vi "ReadFile.vi"(11 "UFF Path":path) -> (2 "transfer fct":cluster{"x0":dbl, "df":dbl, dbl[]}[](graph))   [LabVIEW 2024]
uses:
  PreferencesControl.ctl
panel:
  out "Header Info":T1
  out "Y":cdb[](array[numeric])
  out "Info 3":T2 {"Sampling Type" items=["Dynamic", "Static", "RPM from Tach", "Freq from Tach"]; "Z-axis Data Type Qualifier" items=["Translation", "Rotation", "Translation squared", "Rotation squared"]; "Ordinate Denominator Data Type Qualifier" items=["Translation", "Rotation", "Translation squared", "Rotation squared"]; "Ordinate Numerator Data Type Qualifier" items=["Translation", "Rotation", "Translation squared", "Rotation squared"]; "Abscissa Data Type Qualifier" items=["Translation", "Rotation", "Translation squared", "Rotation squared"]; "Normalization Method" items=["Unknown", "Units squared", "Units squared per Hz", "Units squared sec per Hz"]; "Amplitude units" items=["unknown", "Half-peak scale", "Peak scale", "RMS"]; "Window Type" items=["None", "Hanning Broad", "Hanning Narrow", "Flattop", "Exponential", "Impact", "Impact & Exponential"]; "Weighting Type" items=["None", "A weighting", "B weighting", "C weighting", "D weighting"]}
  out "Info 2":T3 {"Octave Format" items=["Not in octave format", "octave", "/12 octave", "one third octave", "1/n octave"]}
  out "Time n Type":T4={"Date"="Frequency", "Time"="Frequency", "Version from DB"=0.0, "Subversion"=0.0, "File Type"=enum."Universal"}
  out "Last Saved":cluster{"Date":string, "Time":string}={"Date"="Frequency", "Time"="Frequency"}
  out "Parent Program":string="Frequency"
  out "Info":T5
  out "Nodes":T6
  out "Units":T7
  out "Conversions":T8
  out "Data":T9(array[cluster]) {"Data"."dX" format="%#.6f"}
  out "Tracelines":T10 {"nodes defining" items=["move to node", "draw line to node"]}
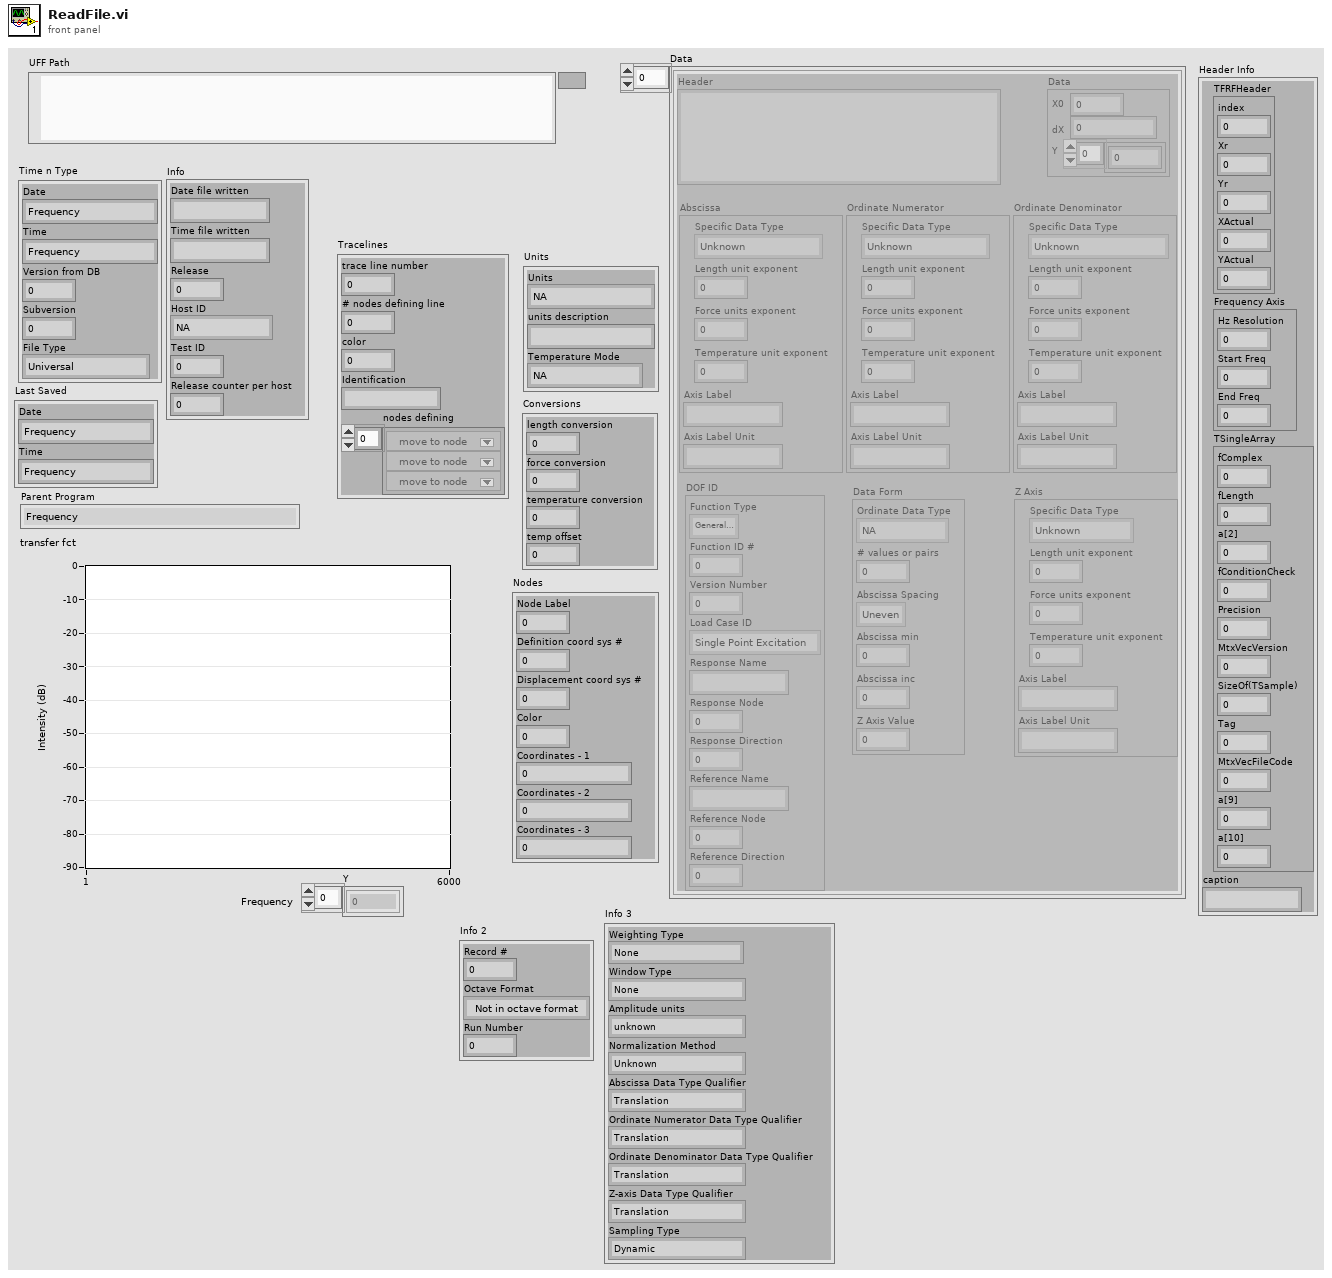
[diagram p1: front panel]
types:
  T1 = cluster{"TFRFHeader":cluster{"index":u32, "Xr":dbl, "Yr":dbl, "XActual":dbl, "YActual":dbl}, "Frequency Axis":cluster{"Hz Resolution":dbl, "Start Freq":dbl, "End Freq":dbl}, "TSingleArray":cluster{"fComplex":u32, "fLength":dbl, "a[2]":dbl, "fConditionCheck":dbl, "Precision":dbl, "MtxVecVersion":dbl, "SizeOf(TSample)":dbl, "Tag":dbl, "MtxVecFileCode":dbl, "a[9]":dbl, "a[10]":dbl}, "caption":string}
  T2 = cluster{"Weighting Type":u16, "Window Type":u16, "Amplitude units":u16, "Normalization Method":u16, "Abscissa Data Type Qualifier":u16, "Ordinate Numerator Data Type Qualifier":u16, "Ordinate Denominator Data Type Qualifier":u16, "Z-axis Data Type Qualifier":u16, "Sampling Type":u16}
  T3 = cluster{"Record #":dbl, "Octave Format":u16, "Run Number":dbl}
  T4 = cluster{"Date":string, "Time":string, "Version from DB":dbl, "Subversion":dbl, "File Type":enum16{"Universal", "Archive", "Other"}}
  T5 = cluster{"Date file written":string, "Time file written":string, "Release":i32, "Host ID":enum16{"NA", "VAX", "SGI", "HP", "RS", "Alp", "Sun", "Sony", "NEC", "Alop/OSF"}, "Test ID":i32, "Release counter per host":i32}
  T6 = cluster{"Node Label":dbl, "Definition coord sys #":dbl, "Displacement coord sys #":dbl, "Color":dbl, "Coordinates - 1":dbl, "Coordinates - 2":dbl, "Coordinates - 3":dbl}
  T7 = cluster{"Units":enum16{"NA", "SIL: Meter", "BG: Foot", "MG: Meter", "BA: Foot", "MM: millimeter", "CM: cm", "IN: inch", "GM: mm", "US: user defined", "MN: mm"}, "units description":string, "Temperature Mode":enum16{"NA", "absolute", "relaitve"}}
  T8 = cluster{"length conversion":dbl, "force conversion":dbl, "temperature conversion":dbl, "temp offset":dbl}
  T9 = cluster{"Abscissa":cluster{"Specific Data Type":enum16{"Unknown", "general", "stress", "strain", "na1", "temperature", "heat flux", "displacement", "na2", "reaction force", "na3", "velocity", "acceleration", "excitation force", "na4", "pressure", "mass", "time", "frequency", "rpm", "order", "sound pressure", "sound intensity", "sound power"}, "Length unit exponent":i32, "Force units exponent":i32, "Temperature unit exponent":i32, "Axis Label":string, "Axis Label Unit":string}, "Ordinate Numerator":cluster{"Specific Data Type":enum16{"Unknown", "general", "stress", "strain", "na1", "temperature", "heat flux", "displacement", "na2", "reaction force", "na3", "velocity", "acceleration", "excitation force", "na4", "pressure", "mass", "time", "frequency", "rpm", "order", "sound pressure", "sound intensity", "sound power"}, "Length unit exponent":i32, "Force units exponent":i32, "Temperature unit exponent":i32, "Axis Label":string, "Axis Label Unit":string}, "Ordinate Denominator":cluster{"Specific Data Type":enum16{"Unknown", "general", "stress", "strain", "na1", "temperature", "heat flux", "displacement", "na2", "reaction force", "na3", "velocity", "acceleration", "excitation force", "na4", "pressure", "mass", "time", "frequency", "rpm", "order", "sound pressure", "sound intensity", "sound power"}, "Length unit exponent":i32, "Force units exponent":i32, "Temperature unit exponent":i32, "Axis Label":string, "Axis Label Unit":string}, "Z Axis":cluster{"Specific Data Type":enum16{"Unknown", "general", "stress", "strain", "na1", "temperature", "heat flux", "displacement", "na2", "reaction force", "na3", "velocity", "acceleration", "excitation force", "na4", "pressure", "mass", "time", "frequency", "rpm", "order", "sound pressure", "sound intensity", "sound power"}, "Length unit exponent":i32, "Force units exponent":i32, "Temperature unit exponent":i32, "Axis Label":string, "Axis Label Unit":string}, "Data Form":cluster{"Ordinate Data Type":enum16{"NA", "NA2", "Real SGL", "NA3", "Real DBL", "Complex SGL", "Complex DBL"}, "# values or pairs":i32, "Abscissa Spacing":enum16{"Uneven", "Even"}, "Abscissa min":dbl, "Abscissa inc":dbl, "Z Axis Value":dbl}, "DOF ID":cluster{"Function Type":enum16{"General or Unknown", "Time Response", "Auto Spectrum", "Cross Spectrum", "FRF", "Transmissibility", "Coherence", "Auto Correlation", "Cross Correlation", "Power Spectral Density", "Energy Spectral Density Function", "Prob Density Function", "Spectrum", "Cumulative Freq Dist", "Peaks Valley", "Stress/Cycles", "Strain/Cycles", "Orbit", "Mode Indicator Funct", "Force Pattern", "Partial Power", "Partial Coherence", "Eigenvalue", "Eigenvector", "Shock Response Spectrum", "Finite Inpulse Response Filter", "Multiple Coherence", "Order Function", "Phase Compensation"}, "Function ID #":i32, "Version Number":i32, "Load Case ID":enum16{"Single Point Excitation"}, "Response Name":string, "Response Node":i32, "Response Direction":i8, "Reference Name":string, "Reference Node":i32, "Reference Direction":i8}, "Data":cluster{"X0":dbl, "dX":dbl, "Y":dbl[]}, "Header":string}[]
  T10 = cluster{"trace line number":i16, "# nodes defining line":i16, "color":i16, "Identification":string, "nodes defining":u16[]}
  T11 = typedef "PreferencesControl.ctl" = cluster{"Name of test":string, "Date":timestamp, "Location":string, "Template":string, "Soundcard":string, "resolution":u16, "Sampling rate":u16, "Ch1 Gain ":dbl, "Ch2 Gain":dbl, "Sample time (s)":dbl, "Pre-trigger (s)":dbl, "Hammer Threshold":dbl, "Positions":i16, "Taps/Position":i16, "Set Names":string, "Freq resolution":dbl, "Hammer cutoff":dbl, "Mic cutoff":dbl, "Double bounce ":dbl, "Hammer Cal":dbl, "dB Offset":dbl, "Accel Cal":dbl, "Vibrometer Cal":dbl, "Mic Cal":dbl, "Output":u16, "Voltage Cal":dbl, "Vibrometer Port":refnum<visa-resource-name>, "Range":u16, "High Pass":u16, "Bandwidth":u16, "X Range":cluster{"Minimum":dbl, "Maximum":dbl, "Increment":dbl, "Minor Increment":dbl, "Start":dbl}[], "Y Range":cluster{"Minimum":dbl, "Maximum":dbl, "Increment":dbl, "Minor Increment":dbl, "Start":dbl}[], "dB Spread":dbl, "Trigger":u16, "Ch_1":u8, "Ch_2":u8, "flip?":bool, "60Hz":bool, "Time offset":dbl, "Piezo Cal":dbl, "Default Notes":string}
  T12 = cluster{"Abscissa":cluster{"Specific Data Type":enum16{"Unknown", "general", "stress", "strain", "na1", "temperature", "heat flux", "displacement", "na2", "reaction force", "na3", "velocity", "acceleration", "excitation force", "na4", "pressure", "mass", "time", "frequency", "rpm", "order", "sound pressure", "sound intensity", "sound power"}, "Length unit exponent":i32, "Force units exponent":i32, "Temperature unit exponent":i32, "Axis Label":string, "Axis Label Unit":string}, "Ordinate Numerator":cluster{"Specific Data Type":enum16{"Unknown", "general", "stress", "strain", "na1", "temperature", "heat flux", "displacement", "na2", "reaction force", "na3", "velocity", "acceleration", "excitation force", "na4", "pressure", "mass", "time", "frequency", "rpm", "order", "sound pressure", "sound intensity", "sound power"}, "Length unit exponent":i32, "Force units exponent":i32, "Temperature unit exponent":i32, "Axis Label":string, "Axis Label Unit":string}, "Ordinate Denominator":cluster{"Specific Data Type":enum16{"Unknown", "general", "stress", "strain", "na1", "temperature", "heat flux", "displacement", "na2", "reaction force", "na3", "velocity", "acceleration", "excitation force", "na4", "pressure", "mass", "time", "frequency", "rpm", "order", "sound pressure", "sound intensity", "sound power"}, "Length unit exponent":i32, "Force units exponent":i32, "Temperature unit exponent":i32, "Axis Label":string, "Axis Label Unit":string}, "Z Axis":cluster{"Specific Data Type":enum16{"Unknown", "general", "stress", "strain", "na1", "temperature", "heat flux", "displacement", "na2", "reaction force", "na3", "velocity", "acceleration", "excitation force", "na4", "pressure", "mass", "time", "frequency", "rpm", "order", "sound pressure", "sound intensity", "sound power"}, "Length unit exponent":i32, "Force units exponent":i32, "Temperature unit exponent":i32, "Axis Label":string, "Axis Label Unit":string}, "Data Form":cluster{"Ordinate Data Type":enum16{"NA", "NA2", "Real SGL", "NA3", "Real DBL", "Complex SGL", "Complex DBL"}, "# values or pairs":i32, "Abscissa Spacing":enum16{"Uneven", "Even"}, "Abscissa min":dbl, "Abscissa inc":dbl, "Z Axis Value":dbl}, "DOF ID":cluster{"Function Type":enum16{"General or Unknown", "Time Response", "Auto Spectrum", "Cross Spectrum", "FRF", "Transmissibility", "Coherence", "Auto Correlation", "Cross Correlation", "Power Spectral Density", "Energy Spectral Density Function", "Prob Density Function", "Spectrum", "Cumulative Freq Dist", "Peaks Valley", "Stress/Cycles", "Strain/Cycles", "Orbit", "Mode Indicator Funct", "Force Pattern", "Partial Power", "Partial Coherence", "Eigenvalue", "Eigenvector", "Shock Response Spectrum", "Finite Inpulse Response Filter", "Multiple Coherence", "Order Function", "Phase Compensation"}, "Function ID #":i32, "Version Number":i32, "Load Case ID":enum16{"Single Point Excitation"}, "Response Name":string, "Response Node":i32, "Response Direction":i8, "Reference Name":string, "Reference Node":i32, "Reference Direction":i8}, "Data":cluster{dbl, dbl, dbl[]}, "Header":string}[]
  T13 = cluster{"Abscissa":cluster{"Specific Data Type":enum16{"Unknown", "general", "stress", "strain", "na1", "temperature", "heat flux", "displacement", "na2", "reaction force", "na3", "velocity", "acceleration", "excitation force", "na4", "pressure", "mass", "time", "frequency", "rpm", "order", "sound pressure", "sound intensity", "sound power"}, "Length unit exponent":i32, "Force units exponent":i32, "Temperature unit exponent":i32, "Axis Label":string, "Axis Label Unit":string}, "Ordinate Numerator":cluster{"Specific Data Type":enum16{"Unknown", "general", "stress", "strain", "na1", "temperature", "heat flux", "displacement", "na2", "reaction force", "na3", "velocity", "acceleration", "excitation force", "na4", "pressure", "mass", "time", "frequency", "rpm", "order", "sound pressure", "sound intensity", "sound power"}, "Length unit exponent":i32, "Force units exponent":i32, "Temperature unit exponent":i32, "Axis Label":string, "Axis Label Unit":string}, "Ordinate Denominator":cluster{"Specific Data Type":enum16{"Unknown", "general", "stress", "strain", "na1", "temperature", "heat flux", "displacement", "na2", "reaction force", "na3", "velocity", "acceleration", "excitation force", "na4", "pressure", "mass", "time", "frequency", "rpm", "order", "sound pressure", "sound intensity", "sound power"}, "Length unit exponent":i32, "Force units exponent":i32, "Temperature unit exponent":i32, "Axis Label":string, "Axis Label Unit":string}, "Z Axis":cluster{"Specific Data Type":enum16{"Unknown", "general", "stress", "strain", "na1", "temperature", "heat flux", "displacement", "na2", "reaction force", "na3", "velocity", "acceleration", "excitation force", "na4", "pressure", "mass", "time", "frequency", "rpm", "order", "sound pressure", "sound intensity", "sound power"}, "Length unit exponent":i32, "Force units exponent":i32, "Temperature unit exponent":i32, "Axis Label":string, "Axis Label Unit":string}, "Data Form":cluster{"Ordinate Data Type":enum16{"NA", "NA2", "Real SGL", "NA3", "Real DBL", "Complex SGL", "Complex DBL"}, "# values or pairs":i32, "Abscissa Spacing":enum16{"Uneven", "Even"}, "Abscissa min":dbl, "Abscissa inc":dbl, "Z Axis Value":dbl}, "DOF ID":cluster{"Function Type":enum16{"General or Unknown", "Time Response", "Auto Spectrum", "Cross Spectrum", "FRF", "Transmissibility", "Coherence", "Auto Correlation", "Cross Correlation", "Power Spectral Density", "Energy Spectral Density Function", "Prob Density Function", "Spectrum", "Cumulative Freq Dist", "Peaks Valley", "Stress/Cycles", "Strain/Cycles", "Orbit", "Mode Indicator Funct", "Force Pattern", "Partial Power", "Partial Coherence", "Eigenvalue", "Eigenvector", "Shock Response Spectrum", "Finite Inpulse Response Filter", "Multiple Coherence", "Order Function", "Phase Compensation"}, "Function ID #":i32, "Version Number":i32, "Load Case ID":enum16{"Single Point Excitation"}, "Response Name":string, "Response Node":i32, "Response Direction":i8, "Reference Name":string, "Reference Node":i32, "Reference Direction":i8}, "Data":cluster{dbl, dbl, dbl[]}, "Header":string}
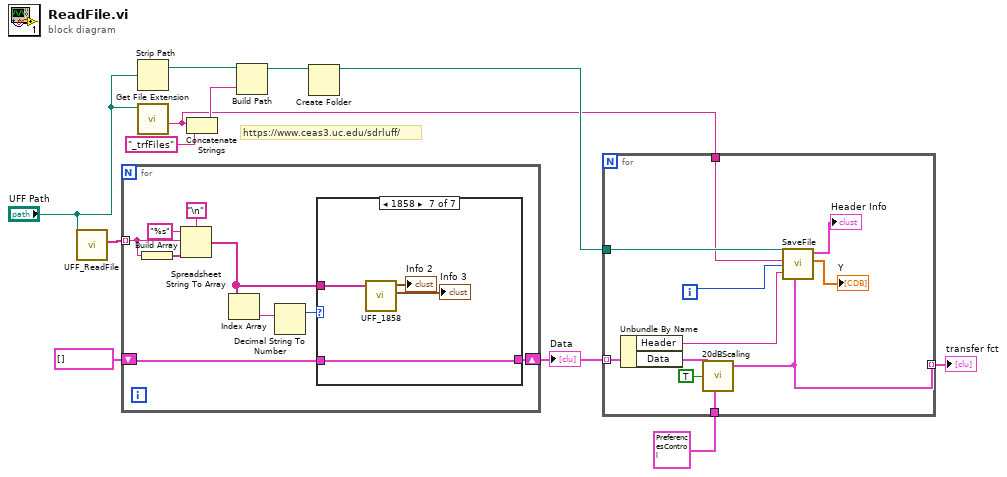
[diagram p0: block diagram]
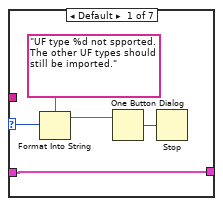
[diagram p2: hidden frame]
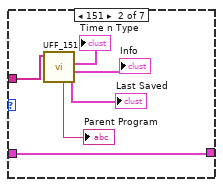
[diagram p3: hidden frame]
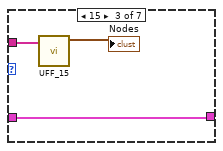
[diagram p4: hidden frame]
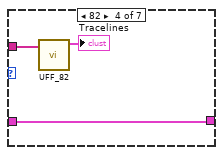
[diagram p5: hidden frame]
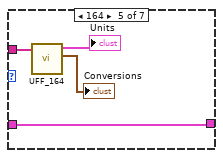
[diagram p6: hidden frame]
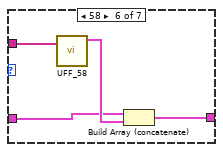
[diagram p7: hidden frame]
diagram:
  # "https://www.ceas3.uc.edu/sdrluff/"
  n1 = call "UFF_ReadFile.vi"("file (use dialog)"="UFF Path") -> ("packets"=w10:string[])  [unwired: 9 in, 1 out]
  n2 = for {
    tunnel: w10 -> [w18] mode=indexing
    shift-right: [w14] -> w11
    shift-left: T12 [] -> [w13]
    n3 = Build Array(w18) -> (w21:string[])
    n4 = Spreadsheet String To Array(delimiter (Tab)="\n", format string="%s", spreadsheet string=w18, array type (2D Dbl)=w21) -> (array=w16:string[])
    n5 = Index Array(array=w16) -> (element=w15:string)  [unwired: 1 in]
    n6 = Decimal String To Number(string=w15) -> (number=w17:i32)  [unwired: 2 in, 1 out]
    n7 = case shown="1858" w17 {
      selector: w17 -> [w25 _ _ _ _ _ _]
      tunnel: w16 -> [_ w32 w35 w38 w42 w46 w50]
      tunnel: [w26 w27 w33 w37 w39 w44 w49] -> w14
      tunnel: w13 -> [w26 w27 w33 w37 w39 w43 w49]
      frame Default {
        n8 = Format Into String(format string="UF type %d not spported.  The other UF types should still be imported.", w25) -> (resulting string=w23:string)  [unwired: 2 in, 1 out]
        n9 = One Button Dialog(message=w23) -> (true=w22:bool)  [unwired: 1 in]
        n10 = Stop(stop? (T)=w22) -> ()
      }
      frame 151 {
        n11 = call "UFF_151.vi"("array"=w32) -> ("Last Saved"=→"Last Saved":cluster{"Date":string, "Time":string}, "Info"=→"Info":T5, "Time n Type"=→"Time n Type":T4, "Parent Program"=→"Parent Program":string)  [unwired: 6 in, 1 out]
      }
      frame 15 {
        n12 = call "UFF_15.vi"("array"=w35) -> ("Nodes"=→"Nodes":T6)  [unwired: 10 in]
      }
      frame 82 {
        n13 = call "UFF_82.vi"("array"=w38) -> ("Tracelines"=→"Tracelines":T10)  [unwired: 10 in]
      }
      frame 164 {
        n14 = call "UFF_164.vi"("array"=w42) -> ("Conversions"=→"Conversions":T8, "Units"=→"Units":T7)  [unwired: 9 in]
      }
      frame 58 {
        n15 = call "UFF_58.vi"("array"=w46) -> ("DataSet"=w45:T13)  [unwired: 10 in]
        n16 = Build Array (concatenate)(w43, w45) -> (w44:T12)
      }
      frame 1858 {
        n17 = call "UFF_1858.vi"("array"=w50) -> ("Hreaders"=→"Info 3":T2, "Info"=→"Info 2":T3)  [unwired: 9 in]
      }
    }
  }
  "Data" <- w11
  n18 = Strip Path(path="UFF Path") -> (stripped path=w7:path)  [unwired: 1 out]
  n19 = call <vilib>:"Get File Extension.vi"("file"="UFF Path") -> ("filename without extension"=w1:string)  [unwired: 6 in, 4 out]
  n20 = Concatenate Strings(w1, "_trfFiles" ("string")) -> (w2:string)
  n21 = Build Path(base path=w7, name or relative path=w2) -> (appended path=w6:path)
  n22 = Create Folder(path (use dialog)=w6) -> (created path=w5:path)  [unwired: 2 in, 2 out]
  n23 = for {
    tunnel: w11 -> [w61] mode=indexing
    tunnel: T11 {"Name of test"="", "Date"=timestamp(0 s since 1904-01-01), "Location"="", "Template"="", "Soundcard"="", "resolution"=32, "Sampling rate"=48000, "Ch1 Gain "=25.0, "Ch2 Gain"=10.0, "Sample time (s)"=0.3, "Pre-trigger (s)"=0.01, "Hammer Threshold"=10.0, "Positions"=12, "Taps/Position"=5, "Set Names"="", "Freq resolution"=10.0, "Hammer cutoff"=0.0, "Mic cutoff"=0.0, "Double bounce "=0.0, "Hammer Cal"=10.0, "dB Offset"=0.0, "Accel Cal"=10.0, "Vibrometer Cal"=0.0, "Mic Cal"=0.0, "Output"=2, "Voltage Cal"=1.0, "Vibrometer Port"="ASRL27::INSTR", "Range"=4, "High Pass"=2, "Bandwidth"=4, "X Range"=[], "Y Range"=[], "dB Spread"=0.0, "Trigger"=0, "Ch_1"=25, "Ch_2"=25, "flip?"=FALSE, "60Hz"=FALSE, "Time offset"=0.0, "Piezo Cal"=1.0, "Default Notes"=""} ("Settings in") -> [w59]
    tunnel: [w55] -> w8 mode=indexing
    tunnel: w5 -> [w56]
    tunnel: w1 -> [w51]
    i -> [w54]
    n24 = Unbundle By Name(w61) -> ("Header"=w57:string, "Data"=w58:cluster{dbl, dbl, dbl[]})
    n25 = call "20dBScaling.vi"("Average FRF in"=w58, "dB?"=TRUE, "Settings"=w59) -> ("Average FRF out"=w55:cluster{"x0":dbl, "df":dbl, dbl[]})  [unwired: 3 in, 1 out]
    n26 = call "SaveFile.vi"("Header"=w57, "Average FRF in"=w55, "i"=w54, "filename"=w51, "Folder"=w56) -> ("Y"=→"Y":cdb[], "Header Info"=→"Header Info":T1)  [unwired: 5 in]
  }
  "transfer fct" <- w8
